vi "Obtain Doc Title.vi"(8 "error in (no error)":errorcluster, 11 "Py Shell in":refnum<class "Py Shell.lvclass">) -> (0 "error out":errorcluster, 3 "Py Shell out":refnum<class "Py Shell.lvclass">)   [LabVIEW 2019, in "Py Shell.lvclass"]
uses:
  Py Shell.lvclass
  D:/Namratha/MDI/LabVIEW-MDI-develop_LV2019/source code/Document/Py Doc/Py Doc.lvclass
  D:/Namratha/MDI/LabVIEW-MDI-develop_LV2019/source code/Document/Document base/Document.lvclass
  Document base/Document.lvclass/Document.ctl
  Property/Read Py File Path.vi
  Document base/property/Write Doc Title.vi
  <vilib>/regexp/Match Regular Expression.xnode
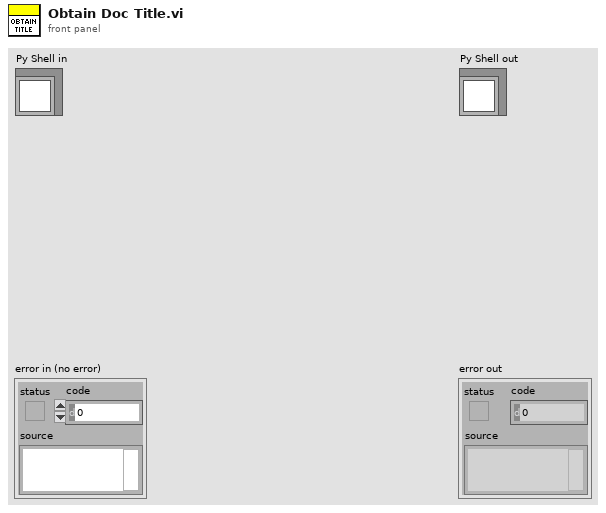
[diagram p1: front panel]
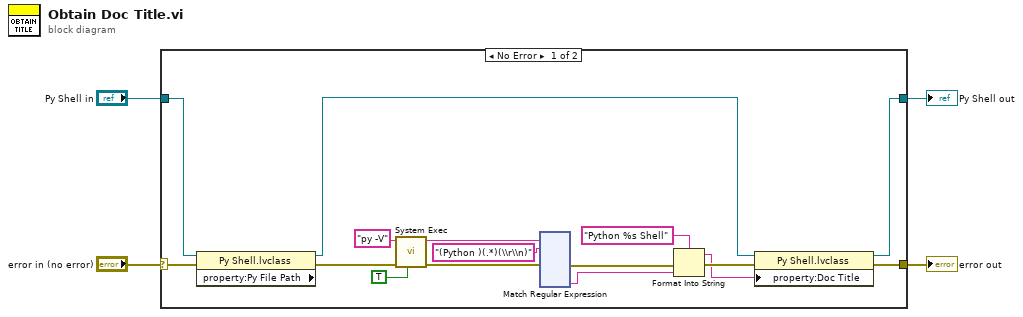
[diagram p0: block diagram]
diagram:
  n1 = case shown="No Error" "error in (no error)" {
    selector: "error in (no error)" -> [w20 w138]
    tunnel: "Py Shell in" -> [w19 w139]
    tunnel: [w16 w139] -> w3
    tunnel: [w18 w138] -> w1
    frame No Error {
      n2 = property class="Py Shell.lvclass" props=["property:Py File Path"](reference=w19, error in=w20) -> (reference out=w17:refnum<class "Py Shell.lvclass">, error out=w7:errorcluster)  [unwired: 1 out]
      n3 = call <vilib>:"System Exec.vi"("run minimized? (F)"=TRUE, "error in (no error)"=w7, "command line"="py -V") -> ("error out"=w9:errorcluster, "standard output"=w10:string)  [unwired: 5 in, 2 out]
      n4 = xnode "Match Regular Expression"("input string"=w10, "regular expression"="(Python )(.*)(\\r\\n)", "error in"=w9) -> ("error out"=w15:errorcluster, "submatch 2"=w13:string)  [unwired: 3 in, 5 out]
      n5 = Format Into String(format string="Python %s Shell", error in=w15, w13) -> (resulting string=w5:string, error out=w6:errorcluster)  [unwired: 1 in]
      n6 = property class="Py Shell.lvclass"(reference=w17, error in=w6, "property:Doc Title"=w5) -> (reference out=w16:refnum<class "Py Shell.lvclass">, error out=w18:errorcluster)
    }
    frame Error {
    }
  }
  "error out" <- w1
  "Py Shell out" <- w3
